vi "CalculateFixedPlusRandom2.vi"(3 "Component times":cluster{"Fixed (s)":dbl, "Random (s)":dbl}={"Fixed (s)"=0.0, "Random (s)"=2.0} {"Random (s)" format="%.4f"; "Fixed (s)" format="%_4g"}) -> (0 "time in ms":dbl, 1 "Composite time":dbl format="%.4f")   [LabVIEW 2010]
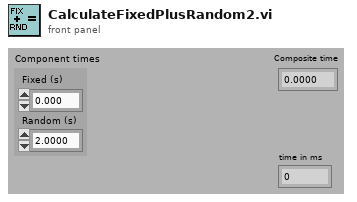
[diagram p1: front panel]
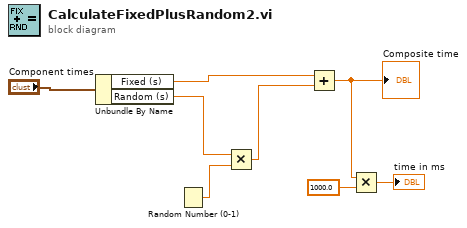
[diagram p0: block diagram]
diagram:
  n1 = Unbundle By Name("Component times") -> ("Fixed (s)"=w5:dbl, "Random (s)"=w4:dbl)
  n2 = Random Number (0-1)() -> (number: 0 to 1=w8:dbl)
  n3 = Multiply(x=w4, y=w8) -> (x*y=w7:dbl)
  n4 = Add(x=w5, y=w7) -> (x+y=w3:dbl)
  "Composite time" <- w3
  n5 = Multiply(x=w3, y=1000.0) -> (x*y=→"time in ms":dbl)
